vi "TermLoopBack-old.vi"(0 "VISA resource name":refnum<visa-resource-name>="COM1", 1 "error in (no error)":errorcluster {"code" format="%.0x"}) -> (2 "VISA resource name Out":refnum<visa-resource-name>, 3 "Receive_buffer":u8[](array[numeric]) format="%x", 4 "error out":errorcluster)   [LabVIEW 2014]
uses:
  <instrlib>/niSwitch/niswitch.llb/niSwitch Topologies.ctl
panel:
  in  "topology name":T1="2566/16-SPDT"
  in  "resource name":refnum<k15>="PXI1Slot6"
  out "Read Count":u32
  out "Write Count":u32
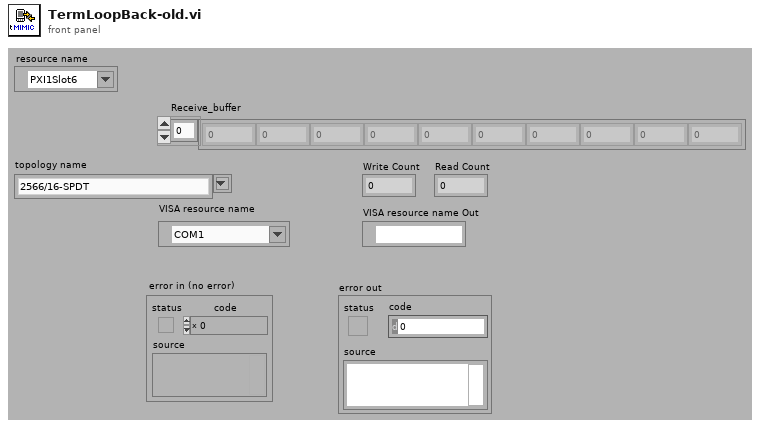
[diagram p1: front panel]
types:
  T1 = typedef "niSwitch Topologies.ctl" = string
  T2 = enum16{"Init Control Relays", "Secondary RS232", "Term Loopback", "CTS Isolate", "Synapse Loopback", "CST RTS Loopback", "Command Flash", "Auxillary RS232", "Battery Charge", "Remote Power", "Cordless Boot", "Auxillary Port", "DeInit Control Relays"}
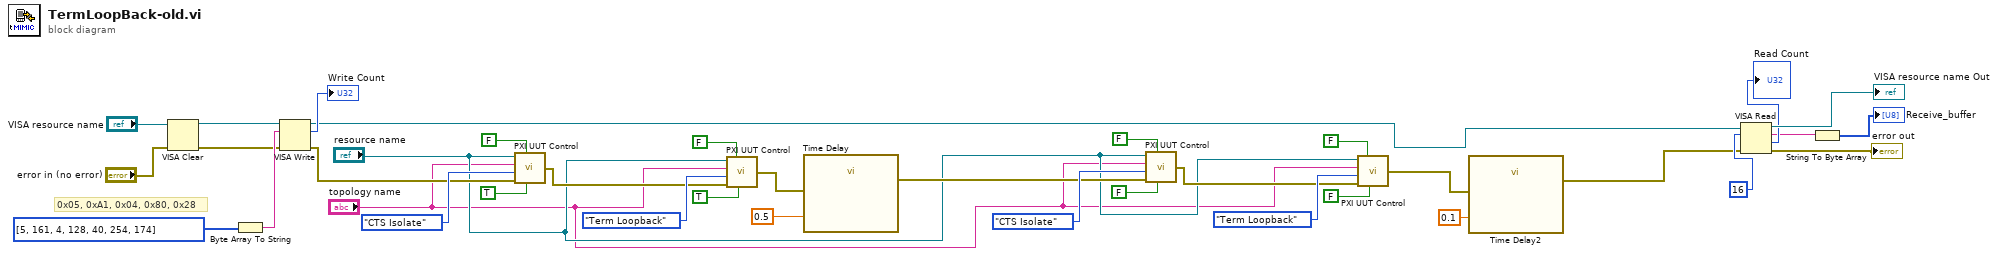
[diagram p0: block diagram]
diagram:
  # "0x05, 0xA1, 0x04, 0x80, 0x28"
  n1 = VISA Clear(VISA resource name="VISA resource name", error in (no error)="error in (no error)") -> (VISA resource name out=w25:refnum<visa-resource-name>, error out=w24:errorcluster)
  n2 = Byte Array To String(unsigned byte array=u8[] [5, 161, 4, 128, 40, 254, 174] ("Command array")) -> (string=w35:string)
  n3 = VISA Write(VISA resource name=w25, write buffer=w35, error in (no error)=w24) -> (VISA resource name out=w1:refnum<visa-resource-name>, return count=→"Write Count":u32, error out=w18:errorcluster)
  n4 = call "PXI UUT Control.vi"("Enable Relays"=TRUE, "Reset IO"=FALSE, "error in (no error)"=w18, "Enum"=T2."CTS Isolate", "topology name"="topology name", "resource name"="resource name") -> ("error out"=w16:errorcluster)
  n5 = call "PXI UUT Control.vi"("Enable Relays"=TRUE, "Reset IO"=FALSE, "error in (no error)"=w16, "Enum"=T2."Term Loopback", "topology name"="topology name", "resource name"="resource name") -> ("error out"=w15:errorcluster)
  n6 = call "Time Delay"("error in (no error)"=w15, "Delay Time (s)"=0.5) -> ("error out"=w6:errorcluster)  [unwired: 9 in]
  n7 = call "PXI UUT Control.vi"("Enable Relays"=FALSE, "Reset IO"=FALSE, "error in (no error)"=w6, "Enum"=T2."CTS Isolate", "topology name"="topology name", "resource name"="resource name") -> ("error out"=w7:errorcluster)
  n8 = call "PXI UUT Control.vi"("Enable Relays"=FALSE, "Reset IO"=FALSE, "error in (no error)"=w7, "Enum"=T2."Term Loopback", "topology name"="topology name", "resource name"="resource name") -> ("error out"=w2:errorcluster)
  n9 = call "Time Delay2"("error in (no error)"=w2, "Delay Time (s)"=0.1) -> ("error out"=w3:errorcluster)  [unwired: 9 in]
  n10 = VISA Read(VISA resource name=w1, byte count=u32 16, error in (no error)=w3) -> (VISA resource name out=→"VISA resource name Out":refnum<visa-resource-name>, read buffer=w28:string, return count=→"Read Count":u32, error out=→"error out":errorcluster)
  n11 = String To Byte Array(string=w28) -> (unsigned byte array=→"Receive_buffer":u8[])
